vi "Codec_CMD_1.vi"(6 "F/T-B":cluster{"Rack":string, "DUT Status":string[]}[](array[cluster])=[{"Rack"="101", "DUT Status"=["READY", "READY", "READY", "READY", "READY"]}, {"Rack"="102", "DUT Status"=["READY", "READY", "READY", "READY", "READY"]}], 8 "error in (no error)":errorcluster, 9 "F/T":cluster{"Rack":string, "DUT Status":string[]}[](array[cluster])=[{"Rack"="201", "DUT Status"=["READY", "READY", "READY", "READY", "READY"]}, {"Rack"="202", "DUT Status"=["READY", "READY", "READY", "READY", "READY"]}], 10 "H/P":cluster{"Rack":string, "DUT Status":string[]}[](array[cluster])=[{"Rack"="1", "DUT Status"=["READY"]}], 11 "SecureMqttCodec in":refnum<class "SecureMqttCodec.lvclass">=refnum) -> (0 "error out":errorcluster, 2 "<JSON>":string="{\r  \"CMD\": 1,\r  \"CONTENT\": [\r    {\r      \"COMMAND\": \"SET_SI\",\r      \"F/T\": {\r        \"201\": {\r          \"1\": {\r            \"STATUS\": \"READY\"\r          },\r          \"2\": {\r            \"STATUS\": \"READY\"\r          },\r          \"3\": {\r            \"STATUS\": \"READY\"\r          },\r          \"4\": {\r            \"STATUS\": \"READY\"\r          },\r          \"5\": {\r            \"STATUS\": \"READY\"\r          }\r        },\r        \"202\": {\r          \"1\": {\r            \"STATUS\": \"READY\"\r          },\r          \"2\": {\r            \"STATUS\": \"READY\"\r          },\r          \"3\": {\r            \"STATUS\": \"MAINTAIN\"\r          },\r          \"4\": {\r            \"STATUS\": \"READY\"\r          },\r          \"5\": {\r            \"STATUS\": \"READY\"\r          }\r        },\r        \"203\": {\r          \"1\": {\r            \"STATUS\": \"READY\"\r          },\r          \"2\": {\r            \"STATUS\": \"READY\"\r          },\r          \"3\": {\r            \"STATUS\": \"READY\"\r          },\r          \"4\": {\r            \"STATUS\": \"READY\"\r          },\r          \"5\": {\r            \"STATUS\": \"READY\"\r          }\r        },\r        \"204\": {\r          \"1\": {\r            \"STATUS\": \"READY\"\r          },\r          \"2\": {\r            \"STATUS\": \"READY\"\r          },\r          \"3\": {\r            \"STATUS\": \"READY\"\r          },\r          \"4\": {\r            \"STATUS\": \"READY\"\r          },\r          \"5\": {\r            \"STATUS\": \"READY\"\r          }\r        },\r        \"205\": {\r          \"1\": {\r            \"STATUS\": \"READY\"\r          },\r          \"2\": {\r            \"STATUS\": \"READY\"\r          },\r          \"3\": {\r            \"STATUS\": \"READY\"\r          },\r          \"4\": {\r            \"STATUS\": \"READY\"\r          },\r          \"5\": {\r            \"STATUS\": \"READY\"\r          }\r        },\r        \"206\": {\r          \"1\": {\r            \"STATUS\": \"READY\"\r          },\r          \"2\": {\r            \"STATUS\": \"READY\"\r          },\r          \"3\": {\r            \"STATUS\": \"READY\"\r          },\r          \"4\": {\r            \"STATUS\": \"READY\"\r          },\r          \"5\": {\r            \"STATUS\": \"READY\"\r          }\r        },\r        \"207\": {\r          \"1\": {\r            \"STATUS\": \"READY\"\r          },\r          \"2\": {\r            \"STATUS\": \"READY\"\r          },\r          \"3\": {\r            \"STATUS\": \"READY\"\r          },\r          \"4\": {\r            \"STATUS\": \"READY\"\r          },\r          \"5\": {\r            \"STATUS\": \"READY\"\r          }\r        },\r        \"208\": {\r          \"1\": {\r            \"STATUS\": \"READY\"\r          },\r          \"2\": {\r            \"STATUS\": \"READY\"\r          },\r          \"3\": {\r            \"STATUS\": \"READY\"\r          },\r          \"4\": {\r            \"STATUS\": \"READY\"\r          },\r          \"5\": {\r            \"STATUS\": \"READY\"\r          }\r        },\r        \"209\": {\r          \"1\": {\r            \"STATUS\": \"READY\"\r          },\r          \"2\": {\r            \"STATUS\": \"READY\"\r          },\r          \"3\": {\r            \"STATUS\": \"READY\"\r          },\r          \"4\": {\r            \"STATUS\": \"READY\"\r          },\r          \"5\": {\r            \"STATUS\": \"READY\"\r          }\r        },\r        \"210\": {\r          \"1\": {\r            \"STATUS\": \"READY\"\r          },\r          \"2\": {\r            \"STATUS\": \"READY\"\r          },\r          \"3\": {\r            \"STATUS\": \"READY\"\r          },\r          \"4\": {\r            \"STATUS\": \"READY\"\r          },\r          \"5\": {\r            \"STATUS\": \"READY\"\r          }\r        },\r        \"211\": {\r          \"1\": {\r            \"STATUS\": \"READY\"\r          },\r          \"2\": {\r            \"STATUS\": \"READY\"\r          },\r          \"3\": {\r            \"STATUS\": \"READY\"\r          },\r          \"4\": {\r            \"STATUS\": \"READY\"\r          },\r          \"5\": {\r            \"STATUS\": \"READY\"\r          }\r        },\r        \"212\": {\r          \"1\": {\r            \"STATUS\": \"READY\"\r          },\r          \"2\": {\r            \"STATUS\": \"READY\"\r          },\r          \"3\": {\r            \"STATUS\": \"READY\"\r          },\r          \"4\": {\r            \"STATUS\": \"READY\"\r          },\r          \"5\": {\r            \"STATUS\": \"READY\"\r          }\r        }\r      },\r      \"F/T-B\": {\r        \"101\": {\r          \"1\": {\r            \"STATUS\": \"READY\"\r          },\r          \"2\": {\r            \"STATUS\": \"READY\"\r          },\r          \"3\": {\r            \"STATUS\": \"READY\"\r          },\r          \"4\": {\r            \"STATUS\": \"READY\"\r          },\r          \"5\": {\r            \"STATUS\": \"READY\"\r          }\r        },\r        \"102\": {\r          \"1\": {\r            \"STATUS\": \"READY\"\r          },\r          \"2\": {\r            \"STATUS\": \"READY\"\r          },\r          \"3\": {\r            \"STATUS\": \"MAINTAIN\"\r          },\r          \"4\": {\r            \"STATUS\": \"READY\"\r          },\r          \"5\": {\r            \"STATUS\": \"READY\"\r          }\r        },\r        \"103\": {\r          \"1\": {\r            \"STATUS\": \"READY\"\r          },\r          \"2\": {\r            \"STATUS\": \"READY\"\r          },\r          \"3\": {\r            \"STATUS\": \"READY\"\r          },\r          \"4\": {\r            \"STATUS\": \"READY\"\r          },\r          \"5\": {\r            \"STATUS\": \"READY\"\r          }\r        },\r        \"104\": {\r          \"1\": {\r            \"STATUS\": \"READY\"\r          },\r          \"2\": {\r            \"STATUS\": \"READY\"\r          },\r          \"3\": {\r            \"STATUS\": \"READY\"\r          },\r          \"4\": {\r            \"STATUS\": \"READY\"\r          },\r          \"5\": {\r            \"STATUS\": \"READY\"\r          }\r        },\r        \"105\": {\r          \"1\": {\r            \"STATUS\": \"READY\"\r          },\r          \"2\": {\r            \"STATUS\": \"READY\"\r          },\r          \"3\": {\r            \"STATUS\": \"READY\"\r          },\r          \"4\": {\r            \"STATUS\": \"READY\"\r          },\r          \"5\": {\r            \"STATUS\": \"READY\"\r          }\r        },\r        \"106\": {\r          \"1\": {\r            \"STATUS\": \"READY\"\r          },\r          \"2\": {\r            \"STATUS\": \"READY\"\r          },\r          \"3\": {\r            \"STATUS\": \"READY\"\r          },\r          \"4\": {\r            \"STATUS\": \"READY\"\r          },\r          \"5\": {\r            \"STATUS\": \"READY\"\r          }\r        },\r        \"107\": {\r          \"1\": {\r            \"STATUS\": \"READY\"\r          },\r          \"2\": {\r            \"STATUS\": \"READY\"\r          },\r          \"3\": {\r            \"STATUS\": \"READY\"\r          },\r          \"4\": {\r            \"STATUS\": \"READY\"\r          },\r          \"5\": {\r            \"STATUS\": \"READY\"\r          }\r        },\r        \"108\": {\r          \"1\": {\r            \"STATUS\": \"READY\"\r          },\r          \"2\": {\r            \"STATUS\": \"READY\"\r          },\r          \"3\": {\r            \"STATUS\": \"READY\"\r          },\r          \"4\": {\r            \"STATUS\": \"READY\"\r          },\r          \"5\": {\r            \"STATUS\": \"READY\"\r          }\r        },\r        \"109\": {\r          \"1\": {\r            \"STATUS\": \"READY\"\r          },\r          \"2\": {\r            \"STATUS\": \"READY\"\r          },\r          \"3\": {\r            \"STATUS\": \"READY\"\r          },\r          \"4\": {\r            \"STATUS\": \"READY\"\r          },\r          \"5\": {\r            \"STATUS\": \"READY\"\r          }\r        },\r        \"110\": {\r          \"1\": {\r            \"STATUS\": \"READY\"\r          },\r          \"2\": {\r            \"STATUS\": \"READY\"\r          },\r          \"3\": {\r            \"STATUS\": \"READY\"\r          },\r          \"4\": {\r            \"STATUS\": \"READY\"\r          },\r          \"5\": {\r            \"STATUS\": \"READY\"\r          }\r        },\r        \"111\": {\r          \"1\": {\r            \"STATUS\": \"READY\"\r          },\r          \"2\": {\r            \"STATUS\": \"READY\"\r          },\r          \"3\": {\r            \"STATUS\": \"READY\"\r          },\r          \"4\": {\r            \"STATUS\": \"READY\"\r          },\r          \"5\": {\r            \"STATUS\": \"READY\"\r          }\r        },\r        \"112\": {\r          \"1\": {\r            \"STATUS\": \"READY\"\r          },\r          \"2\": {\r            \"STATUS\": \"READY\"\r          },\r          \"3\": {\r            \"STATUS\": \"READY\"\r          },\r          \"4\": {\r            \"STATUS\": \"READY\"\r          },\r          \"5\": {\r            \"STATUS\": \"READY\"\r          }\r        }\r      },\r      \"H/P\": {\r        \"1\": {\r          \"1\": {\r            \"STATUS\": \"READY\"\r          }\r        }\r      }\r    }\r  ],\r  \"ERRCODE\": \"\",\r  \"ERRMSG\": \"\",\r  \"FROM\": \"0050C500001E\",\r  \"ID\": \"95D66C2E-6654-4CC1-95AE-F62F0A2E55B4\",\r  \"STATUS\": \"\",\r  \"TIMESTAMP\": 1759399004,\r  \"TO\": \"\"\r}", 3 "SecureMqttCodec out":refnum<class "SecureMqttCodec.lvclass">)   [LabVIEW 2020, in "SecureMqttCodec.lvclass"]
uses:
  SecureMqttCodec.lvclass
  <vilib>/addons/JSON API/JSON Value/JSON Value.lvclass
  <vilib>/addons/JSON API/JSON Object/JSON Object.lvclass
  <vilib>/addons/JSON API/JSON Scalar/JSON Scalar.lvclass
  C:/Program Files/National Instruments/LabVIEW 2020/vi.lib/addons/JSON API/JSON Value/JSON Value.lvclass
  SecureMqttCodec.lvclass/SecureMqttCodec.ctl
  <vilib>/addons/JSON API/JSON Scalar/Set U32.vi
  <vilib>/addons/JSON API/JSON Value/Get as JSON string (pretty).vi
  <vilib>/addons/JSON API/Get Polymorphic/JSON GetSet.lvlib
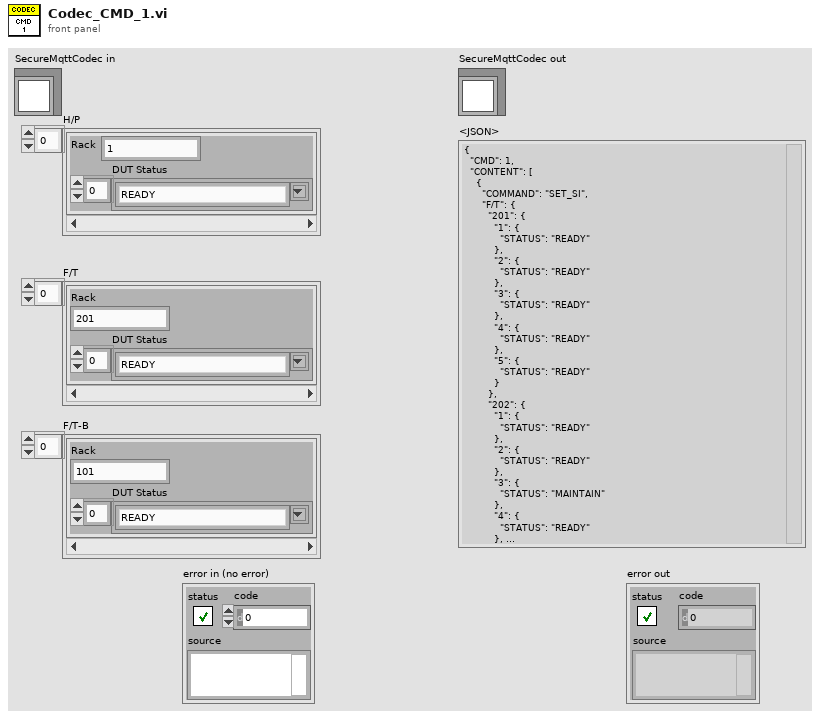
[diagram p1: front panel]
types:
  T1 = cluster{"JsonObj_Ori":refnum<class "JSON Value.lvclass">, "JsonObj_Content":refnum<class "JSON Value.lvclass">, "sJsonOut":string}
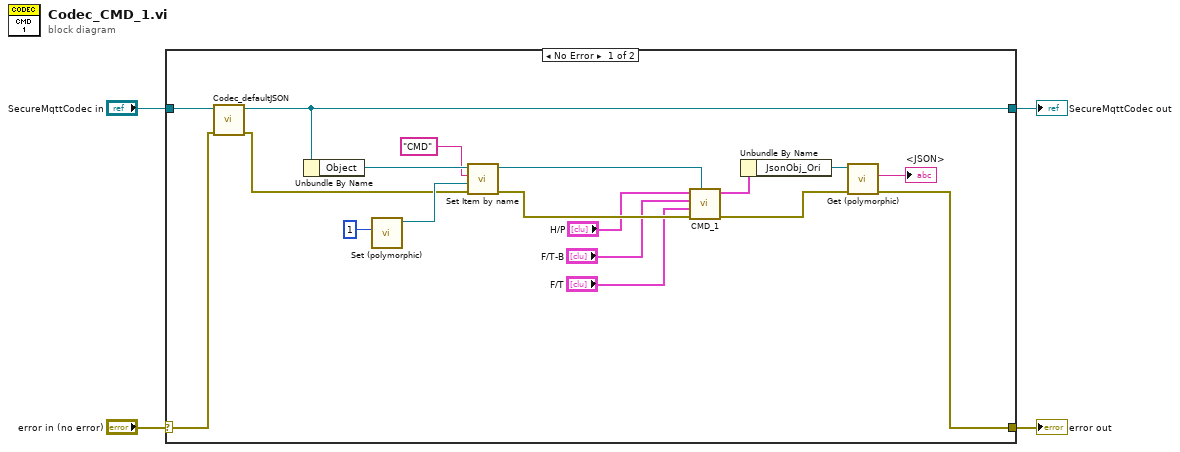
[diagram p0: block diagram]
diagram:
  n1 = case shown="No Error" "error in (no error)" {
    selector: "error in (no error)" -> [w13 w24]
    tunnel: [w18 w24] -> w3
    tunnel: [w16 w23] -> w1
    tunnel: "SecureMqttCodec in" -> [w22 w23]
    frame No Error {
      n2 = call "Codec_defaultJSON.vi"("error in (no error)"=w13, "SecureMqttCodec in"=w22) -> ("error out"=w15:errorcluster, "SecureMqttCodec out"=w16:refnum<class "SecureMqttCodec.lvclass">)  [unwired: 8 in]
      n3 = Unbundle By Name(w16) -> ("Object"=w21:refnum<class "JSON Value.lvclass">)
      n4 = call-poly <vilib>:"Set (polymorphic).vi"("Numeric"=u32 1) -> ("JSON Scalar out"=w19:refnum<class "JSON Scalar.lvclass">)  [unwired: 9 in, 1 out]
      n5 = call-dynamic "Set Item by name.vi"("error in (no error)"=w15, "Value"=w19, "name"="CMD", "JSON Value In"=w21) -> ("error out"=w12:errorcluster, "JSON Value Out"=w11:refnum<class "JSON Value.lvclass">)  [unwired: 5 in, 1 out]
      n6 = call "CMD_1.vi"("JsonObj_Ori"=w11, "error in (no error)"=w12, "F/T"="F/T", "F/T-B"="F/T-B", "H/P"="H/P") -> ("error out"=w8:errorcluster, "Result"=w10:T1)  [unwired: 5 in]
      n7 = Unbundle By Name(w10) -> ("JsonObj_Ori"=w9:refnum<class "JSON Value.lvclass">)
      n8 = call-poly <vilib>:"Get (polymorphic).vi"("error in (no error)"=w8, "JSON Value in"=w9) -> ("error out"=w18:errorcluster, "<JSON>"=→"<JSON>":string)  [unwired: 8 in]
    }
    frame Error {
    }
  }
  "error out" <- w3
  "SecureMqttCodec out" <- w1
